vi "Create Evaluation String.vi"(8 "error in (no error)":errorcluster, 10 "Evaluation String":string, 11 "Str Ends With in":refnum<class "Str Ends With.lvclass">) -> (0 "error out":errorcluster, 3 "Str Ends With out":refnum<class "Str Ends With.lvclass">)   [LabVIEW 2018, in "Str Ends With.lvclass"]
uses:
  Str Ends With.lvclass
  C:/Users/UKHornP/Documents/Work/Projects/Assert_API/Plugins/Utility/Test Classes/Test.lvclass
  String.lvclass
  Test.lvclass
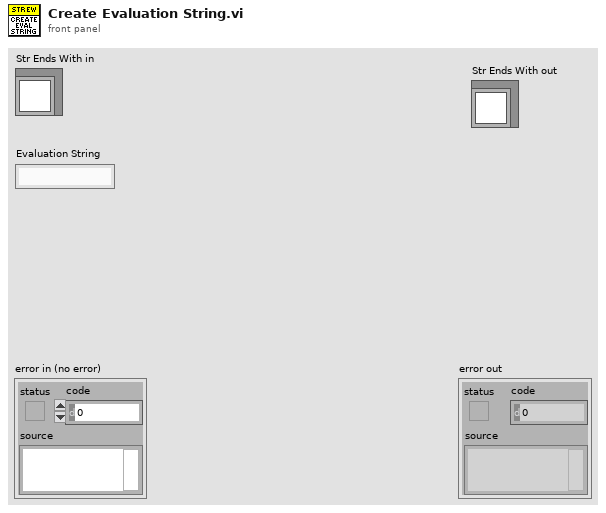
[diagram p1: front panel]
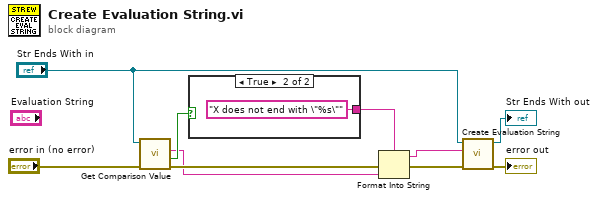
[diagram p0: block diagram]
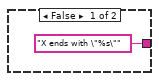
[diagram p2: hidden frame]
diagram:
  n1 = call "Get Comparison Value.vi"("error in (no error)"="error in (no error)", "Test in"="Str Ends With in") -> ("error out"=w8:errorcluster, "Invert Result"=w7:bool, "Data String"=w5:string)  [unwired: 7 in]
  n2 = case shown="True" w7 {
    tunnel: ["X ends with \"%s\"" "X does not end with \"%s\""] -> w6
    frame False {
    }
    frame True {
    }
  }
  n3 = Format Into String(format string=w6, error in=w8, w5) -> (resulting string=w1:string, error out=w4:errorcluster)  [unwired: 1 in]
  n4 = call-parent "Create Evaluation String.vi"("error in (no error)"=w4, "Evaluation String"=w1, "String in"="Str Ends With in") -> ("error out"=→"error out":errorcluster, "String out"=→"Str Ends With out":refnum<class "Str Ends With.lvclass">)  [unwired: 7 in]
